vi "Dispense test - simple.vi"() -> ()   [LabVIEW 2021, in "Test VIs.lvclass"]
uses:
  Test VIs/Test VIs.lvclass
  Classes/Controller/I-O/I-O.lvclass
  Classes/Controller/Controller.lvclass
  Classes/Controller/Dispenser/Dispenser.lvclass
panel:
  out "stop after dispensing":bool
  out "Value":bool
  out "error out":errorcluster
  in  "error in (no error)":errorcluster
  in  "Pressure":i16=20
  in  "Dispense":bool
  in  "stop":bool
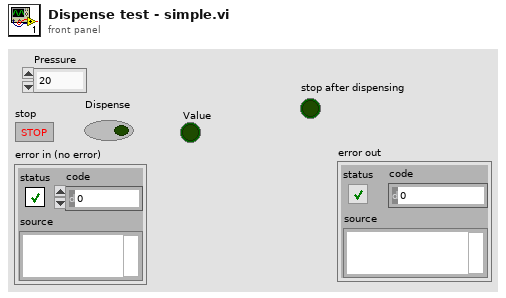
[diagram p1: front panel]
types:
  T1 = typedef "Controller.lvclass/Controllers.ctl" = cluster{"I-O.lvclass":refnum<class "I-O.lvclass">, "Gantry":refnum<k24>, "Dispenser":refnum<visa-resource-name>}
  T2 = typedef "I-O.lvclass/Pin Map.ctl" = cluster{"Region Valves":i32[], "Extra Valves":dbl[][][], "Tool Primary Valve":i32, "Tool Secondary Valve":i32, "Region Sensors":i32[], "Extra Sensors":dbl[][][], "Tool Primary Sensor":dbl, "Tool Secondary Sensor":dbl, "Compression Sensor":dbl, "5V":i32, "Dispenser Sensor":dbl, "Light Curtain":i32}
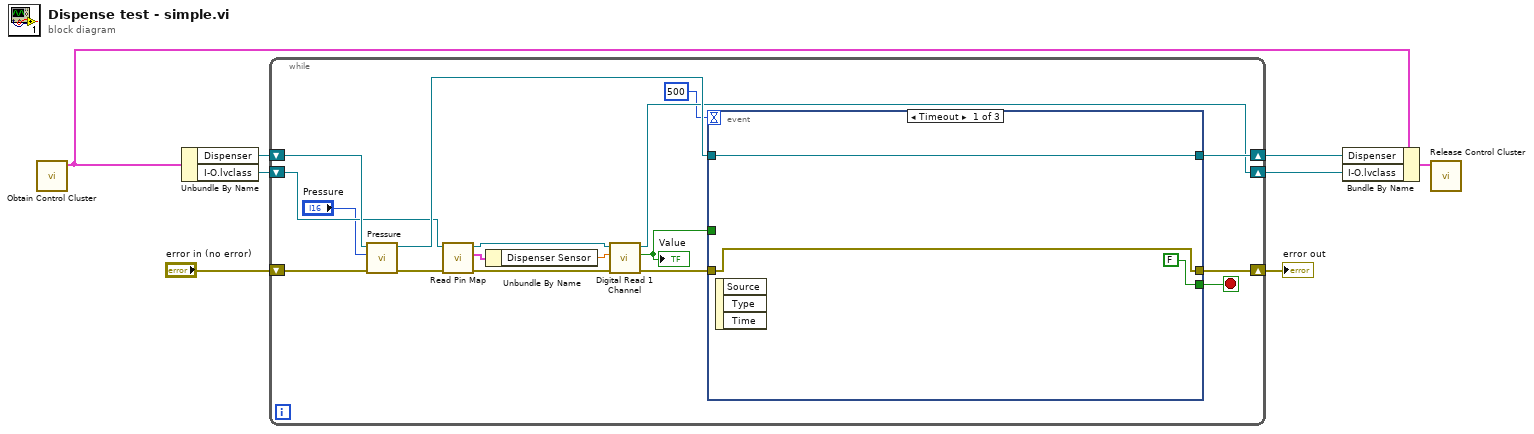
[diagram p0: block diagram]
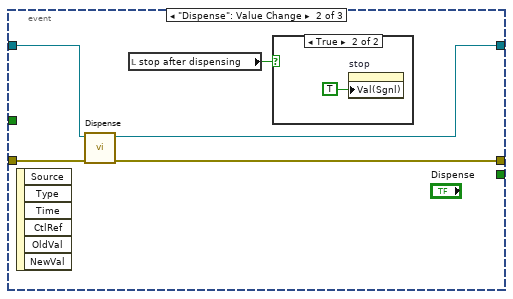
[diagram p2: hidden frame]
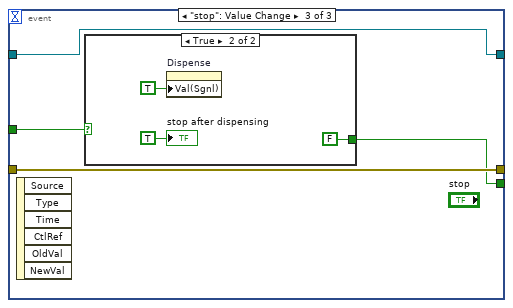
[diagram p4: hidden frame]
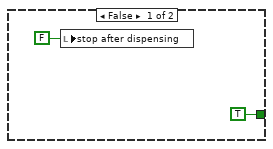
[diagram p5: hidden frame]
diagram:
  n1 = call "Obtain Control Cluster.vi"() -> ("Control Out"=w7:T1)  [unwired: 10 in, 1 out]
  n2 = Unbundle By Name(w7) -> ("Dispenser"=w3:refnum<visa-resource-name>, "I-O.lvclass"=w2:refnum<class "I-O.lvclass">)
  n3 = while {
    shift-right: [w23] -> w5
    shift-left: w3 -> [w22]
    shift-right: [w24] -> w6
    shift-left: "error in (no error)" -> [w18]
    shift-right: [w11] -> w1
    shift-left: w2 -> [w19]
    stop <- w21 stop-if-true
    n4 = call "Pressure.vi"("error in (no error)"=w18, "Pressure"="Pressure", "VISA resource name"=w22) -> ("error out"=w14:errorcluster, "VISA resource name out"=w25:refnum<visa-resource-name>)  [unwired: 7 in]
    n5 = call-dynamic "Read Pin Map.vi"("error in (no error)"=w14, "I-O in"=w19) -> ("error out"=w15:errorcluster, "Pin Map 2"=w20:T2, "I-O out"=w17:refnum<class "I-O.lvclass">)  [unwired: 7 in]
    n6 = Unbundle By Name(w20) -> ("Dispenser Sensor"=w16:dbl)
    n7 = call-dynamic "Digital Read 1 Channel.vi"("error in (no error)"=w15, "Read"=w16, "I-O in"=w17) -> ("error out"=w13:errorcluster, "Value"=w12:bool, "I-O out"=w11:refnum<class "I-O.lvclass">)  [unwired: 6 in]
    "Value" <- w12
    n8 = event shown="[0] Timeout" {
      selector: _ -> [_ _ _]
      dyn-events: _ -> [_ _ _]
      timeout: 500 -> [_ _ _]
      tunnel: w25 -> [w26 w32 w35]
      tunnel: [w26 w30 w35] -> w23
      tunnel: w13 -> [w28 w31 w38]
      tunnel: [w28 w29 w38] -> w24
      tunnel: [FALSE ("stop after dispensing") _ w36] -> w21
      tunnel: w12 -> [_ _ w37]
      event Timeout {
        n9 = event-data() -> ()  [unwired: 1 in, 3 out]
      }
      event "Dispense": Value Change {
        n10 = event-data() -> ()  [unwired: 1 in, 6 out]
        n11 = call "Dispense.vi"("error in (no error)"=w31, "Dispenser In"=w32) -> ("error out"=w29:errorcluster, "Dispenser Out"=w30:refnum<visa-resource-name>)  [unwired: 8 in]
        n12 = local read "stop after dispensing"() -> (w33:bool)
        n13 = case shown="True" w33 {
          frame False {
          }
          frame True {
            n14 = property on="stop" class="Bool (strict)"("Val(Sgnl)"=TRUE ("Value (Signaling)")) -> ()  [unwired: 2 in, 2 out]
          }
        }
      }
      event "stop": Value Change {
        n15 = event-data() -> ()  [unwired: 1 in, 6 out]
        n16 = case shown="True" w37 {
          tunnel: [TRUE FALSE] -> w36
          frame False {
            n17 = local write "stop after dispensing"(FALSE ("stop after dispensing")) -> ()
          }
          frame True {
            n18 = property on="Dispense" class="Bool (strict)"("Val(Sgnl)"=TRUE ("Value (Signaling)")) -> ()  [unwired: 2 in, 2 out]
            "stop after dispensing" <- TRUE ("stop after dispensing")
          }
        }
      }
    }
  }
  "error out" <- w6
  n19 = Bundle By Name(cluster=w7, "Dispenser"=w5, "I-O.lvclass"=w1) -> (w4:T1)
  n20 = call "Release Control Cluster.vi"("output cluster"=w4) -> ()  [unwired: 11 in]
